vi "Destroy Buffer.vi"(8 "error in (no error)":errorcluster, 11 "1D U16 Group With ID DVR Queue in":refnum<class "1D U16 Group With ID DVR Queue.lvclass">) -> (0 "error out":errorcluster, 3 "1D U16 Group With ID DVR Queue out":refnum<class "1D U16 Group With ID DVR Queue.lvclass">)   [LabVIEW 2019, in "1D U16 Group With ID DVR Queue.lvclass"]
uses:
  1D U16 Group With ID DVR Queue.lvclass
  1D U16 Group With ID DVR Queue.lvclass/1D U16 Group With ID DVR Queue.ctl
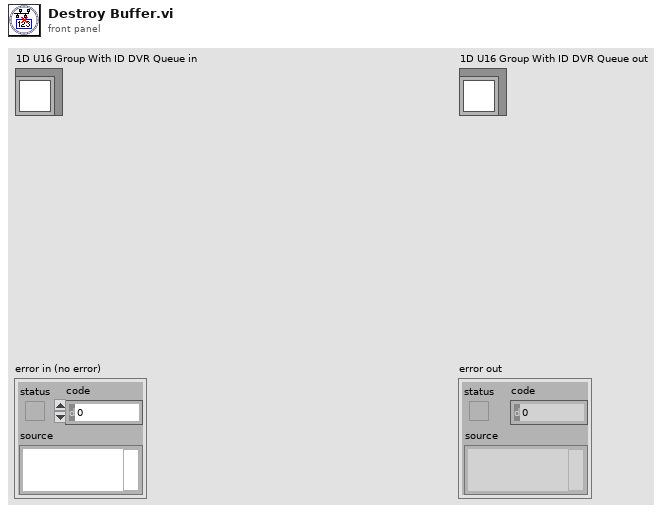
[diagram p1: front panel]
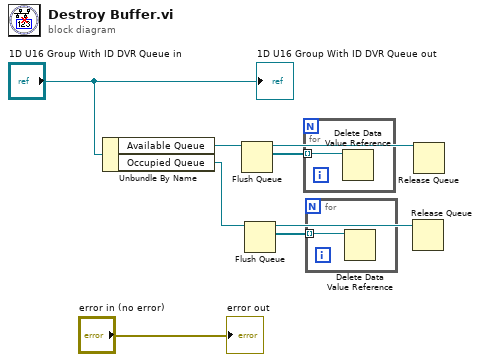
[diagram p0: block diagram]
diagram:
  n1 = Unbundle By Name("1D U16 Group With ID DVR Queue in") -> ("Available Queue"=w7:refnum<queue>, "Occupied Queue"=w6:refnum<queue>)
  n2 = Flush Queue(queue=w7) -> (queue out=w4:refnum<queue>, remaining elements=w5:refnum<data-value>[])  [unwired: 1 in, 1 out]
  n3 = Flush Queue(queue=w6) -> (queue out=w2:refnum<queue>, remaining elements=w3:refnum<data-value>[])  [unwired: 1 in, 1 out]
  n4 = for {
    tunnel: w5 -> [w9] mode=indexing
    n5 = Delete Data Value Reference(data value reference=w9) -> ()  [unwired: 1 in, 2 out]
  }
  n6 = for {
    tunnel: w3 -> [w10] mode=indexing
    n7 = Delete Data Value Reference(data value reference=w10) -> ()  [unwired: 1 in, 2 out]
  }
  n8 = Release Queue(queue=w2) -> ()  [unwired: 2 in, 3 out]
  n9 = Release Queue(queue=w4) -> ()  [unwired: 2 in, 3 out]
  "error out" <- "error in (no error)"
  "1D U16 Group With ID DVR Queue out" <- "1D U16 Group With ID DVR Queue in"
